vi "sub_arrayIntersection.vi"(10 "set 2":string[](array[string]), 11 "set 1":string[](array[string])) -> (3 "set 1  & set 2":string[](array[string]))   [LabVIEW 2018]
panel:
  # "returns the union of set 1 and set 2"
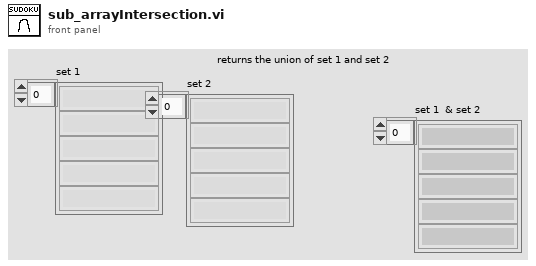
[diagram p1: front panel]
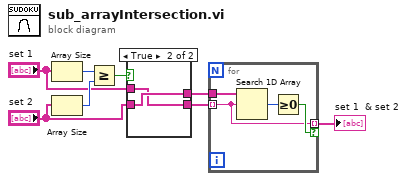
[diagram p0: block diagram]
diagram:
  n1 = Array Size(array="set 1") -> (size(s)=w8:i32)
  n2 = Array Size(array="set 2") -> (size(s)=w7:i32)
  n3 = Greater Or Equal?(x=w8, y=w7) -> (x >= y?=w6:bool)
  n4 = case shown="True" w6 {
    tunnel: "set 1" -> [w10 w11]
    tunnel: [w10 w12] -> w4
    tunnel: "set 2" -> [w9 w12]
    tunnel: [w9 w11] -> w2
    frame False {
    }
    frame True {
    }
  }
  n5 = for {
    tunnel: [w13] -> w1 mode=indexing if=w16
    tunnel: w4 -> [w14]
    tunnel: w2 -> [w13] mode=indexing
    n6 = Search 1D Array(1D array=w14, element=w13) -> (index of element=w15:i32)  [unwired: 1 in]
    n7 = Greater Or Equal To 0?(x=w15) -> (x >= 0?=w16:bool)
  }
  "set 1  & set 2" <- w1
